vi "add delta range(SubVI).vi"(10 "字符串":string) -> (1 "ok or cancel":bool, 2 "连接的字符串":string)   [LabVIEW 2019, in "SubVI.lvlib"]
uses:
  SubVI.lvlib
  lib/Keithley 622x/Configure/2182 -A/Low Level/Typedefs/KE2182 -- Voltage Ranges.ctl
  lib/Keithley 622x/Keithley 622x.lvlib
panel:
  in  "Man / Selected\nRange":T1
  in  "cancel":bool
  in  "ok":bool
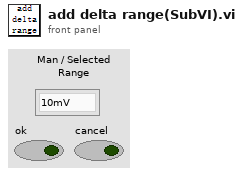
[diagram p1: front panel]
types:
  T1 = typedef "Keithley 622x.lvlib/KE2182 -- Voltage Ranges.ctl" = enum16{"10mV", "100mV", "1V", "10V", "100V"}
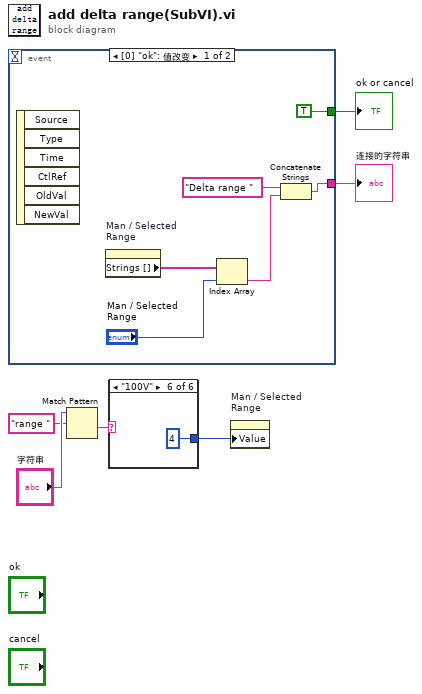
[diagram p0: block diagram]
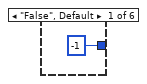
[diagram p2: hidden frame]
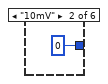
[diagram p3: hidden frame]
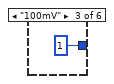
[diagram p4: hidden frame]
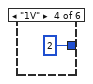
[diagram p5: hidden frame]
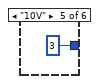
[diagram p6: hidden frame]
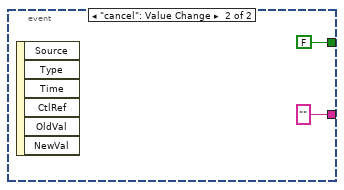
[diagram p7: hidden frame]
diagram:
  n1 = event shown="[0] \"ok\": 值改变" {
    selector: _ -> [_ _]
    dyn-events: _ -> [_ _]
    timeout: _ -> [_ _]
    tunnel: [TRUE FALSE] -> w6
    tunnel: [w10 "" ("分隔符")] -> w5
    event "ok": Value Change {
      n2 = event-data() -> ()  [unwired: 1 in, 6 out]
      n3 = property on="Man / Selected\nRange" class="Enum (严格)"() -> ("Strings []"=w9:string[])  [unwired: 2 in, 2 out]
      n4 = Index Array(array=w9, index="Man / Selected\nRange") -> (element=w7:string)
      n5 = Concatenate Strings("Delta range " ("字符串"), w7) -> (w10:string)
    }
    event "cancel": Value Change {
      n6 = event-data() -> ()  [unwired: 1 in, 6 out]
    }
  }
  "ok or cancel" <- w6
  "连接的字符串" <- w5
  n7 = Match Pattern(string="字符串", regular expression="range ") -> (after substring=w2:string)  [unwired: 1 in, 3 out]
  n8 = case shown="\"100V\"" w2 {
    tunnel: [-1 0 1 2 3 4] -> w1
    frame "False", Default {
    }
    frame "10mV" {
    }
    frame "100mV" {
    }
    frame "1V" {
    }
    frame "10V" {
    }
    frame "100V" {
    }
  }
  n9 = property on="Man / Selected\nRange" class="Enum (严格)"("Value"=w1) -> ()  [unwired: 2 in, 2 out]
